vi "VariantToText.vi"(8 "error in (no error)":errorcluster, 10 "Variant":variant, 11 "BlueJSONTextSerializer in":refnum<class "BlueJSONTextSerializer.lvclass">) -> (0 "error out":errorcluster, 2 "Serializable Text":string, 3 "BlueJSONTextSerializer out":refnum<class "BlueJSONTextSerializer.lvclass">)   [LabVIEW 2019, in "BlueJSONTextSerializer.lvlib" / "BlueJSONTextSerializer.lvclass"]
uses:
  BlueJSONTextSerializer.lvclass
  BlueJSONTextSerializer.lvclass/BlueJSONTextSerializer.ctl
  <vilib>/JDP Science/JSONtext/JSONtext.lvlib
  BlueJSONtext LVClass Serializer/BlueJSONtext LVClass Serializer.lvclass
  C:/Program Files (x86)/National Instruments/LabVIEW 2019/vi.lib/JDP Science/JSONtext/LVClass Serializer/JSONtext LVClass Serializer.lvclass
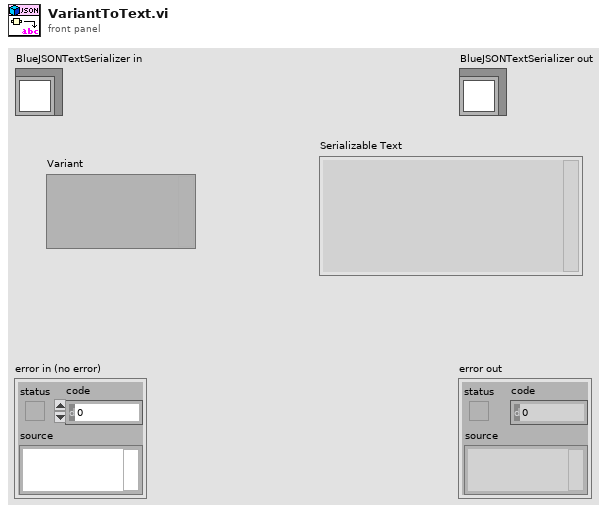
[diagram p1: front panel]
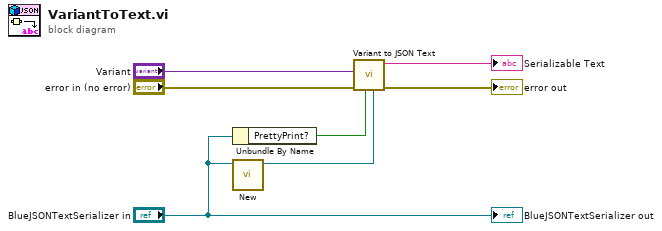
[diagram p0: block diagram]
diagram:
  n1 = Unbundle By Name("BlueJSONTextSerializer in") -> ("PrettyPrint?"=w3:bool)
  n2 = call "New.vi"("BlueJSONTextSerializer"="BlueJSONTextSerializer in") -> ("BlueJSONtext LVClass Serializer out"=w1:refnum<class "BlueJSONtext LVClass Serializer.lvclass">)  [unwired: 10 in]
  n3 = call <vilib>:"Variant to JSON Text.vi"("LVClass Serializer"=w1, "Pretty Print?"=w3, "error in (no error)"="error in (no error)", "Variant"="Variant") -> ("error out"=→"error out":errorcluster, "<JSON>"=→"Serializable Text":string)  [unwired: 5 in, 1 out]
  "BlueJSONTextSerializer out" <- "BlueJSONTextSerializer in"
